vi "kvCanInitialize.vi"(1 "error in (no error)":errorcluster) -> (0 "error out (no error)":errorcluster)   [LabVIEW 2022 SP3]
doc: "This function must be called before any other functions is used. It will initialize the driver. \n\nYou may call canInitializeLibrary more than once. The actual initialization will take place only once. \n\nAny errors encountered during library initialization will be \"silent\" and an appropriate error code will be returned later on when canOpenChannel (or any other API call that requires initialization) is called"
uses:
  canlib32.dll
panel:
  # "This VI has no User Interface.  It simply initializes the KVaser CAN library.  \nOnly the error block is passed through for flow control."
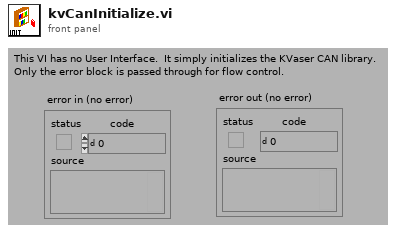
[diagram p1: front panel]
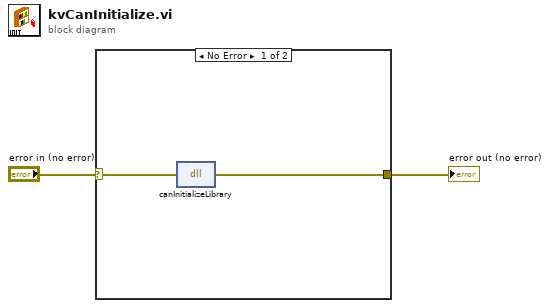
[diagram p0: block diagram]
diagram:
  n1 = case shown="No Error" "error in (no error)" {
    selector: "error in (no error)" -> [w3 w5]
    tunnel: [w4 w5] -> w1
    frame No Error {
      n2 = dll-call lib="canlib32.dll" fn="canInitializeLibrary" label="canInitializeLibrary() Function"(error in=w3) -> (error out=w4:errorcluster)  [unwired: 3 in, 1 out]
    }
    frame Error {
    }
  }
  "error out (no error)" <- w1
